vi "printTSR.vi"(0 "reference in":refnum<class "excelFile.lvclass">, 1 "TSR_details":T1={"Company/Institution:"="", "Address:"="", "Department:"="", "City:"="", "Post Code:"="", "Country:"="", "Contact:"="", "Ref:"="", "Issue description:"="", "Actions:"="", "TYPE:"="Repair", "Shipping:"=0, "Discount:"=0, "dataIN"=[], "Device type:"="microQuark", "Serial Number:"="", "PMC number:"="", "Labour Hours:"=0.0, "Service Location:"=FALSE, "start_hour"="", "end_hour"=""}, 3 "latest_TSR_path":string, 5 "error in (no error)":errorcluster) -> (14 "reference out":refnum<class "excelFile.lvclass">, 17 "PDF_file_path":string, 19 "error out":errorcluster)   [LabVIEW 2015, in "excelFile.lvclass"]
uses:
  excelFile.lvclass
  <vilib>/Utility/error.llb/DialogType.ctl
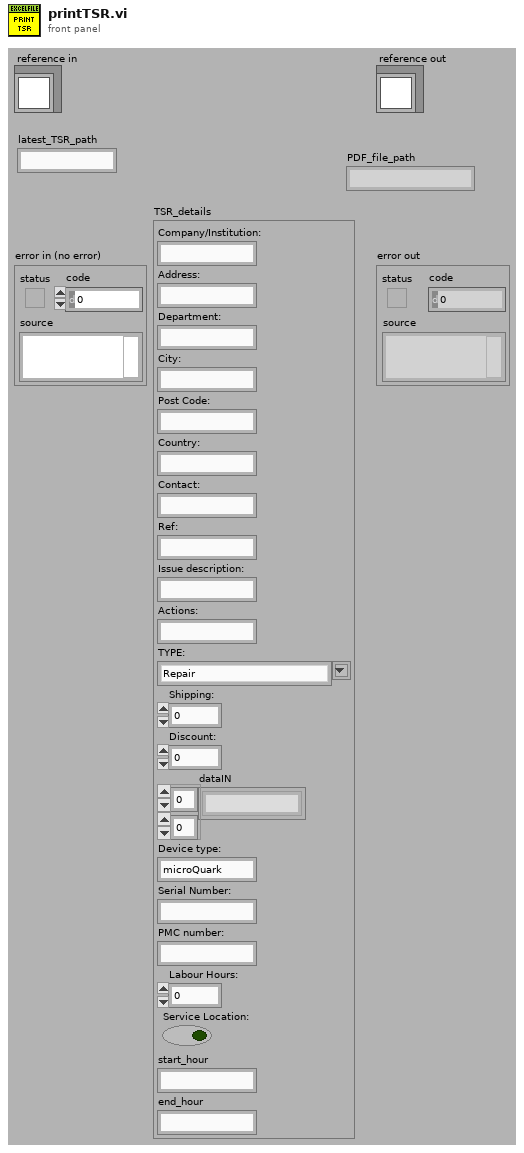
[diagram p1: front panel]
types:
  T1 = cluster{"Company/Institution:":string, "Address:":string, "Department:":string, "City:":string, "Post Code:":string, "Country:":string, "Contact:":string, "Ref:":string, "Issue description:":string, "Actions:":string, "TYPE:":string, "Shipping:":i32, "Discount:":i32, "dataIN":string[][], "Device type:":string, "Serial Number:":string, "PMC number:":string, "Labour Hours:":dbl, "Service Location:":bool, "start_hour":string, "end_hour":string}
  T2 = typedef "excelFile.lvclass/ObjectAttributesRef.ctl" = refnum<data-value>
  T3 = typedef "excelFile.lvclass/ObjectAttributes.ctl" = cluster{"MyAttribute":dbl, "path":string, "Refnum Excel":cluster{"Excel._Application":refnum<k7>, "Workbooks":refnum<k7>, "Open":refnum<k7>}, "data":string[][][], "save":bool, "fileType":T4, "rowsColor":u32[], "python_ref":refnum<class "python.lvclass">, "items_rows":i32[], "excel_range":i32[][], "TSR":cluster{"number":string, "TSR_path":path, "service_path":path, "email_to":string}, "excel_already_opened?":bool, "file_already_opened?":bool, "excel_protected_opened?":bool}
  T4 = typedef "excelFile.lvclass/fileType.ctl" = enum16{"devices", "items", "partsTracking", "TSR"}
  T5 = typedef "DialogType.ctl" = u16
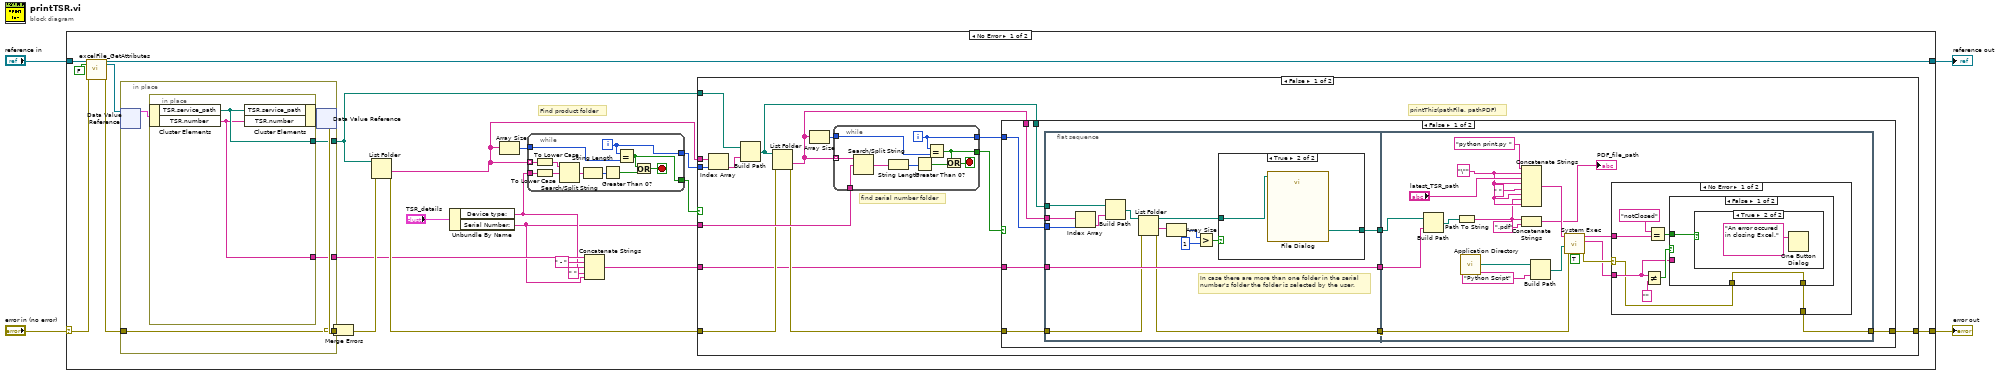
[diagram p0: block diagram]
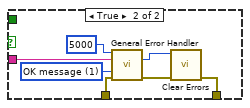
[diagram p4: hidden frame]
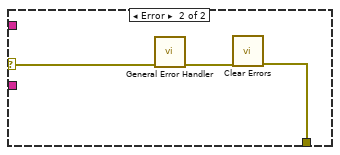
[diagram p5: hidden frame]
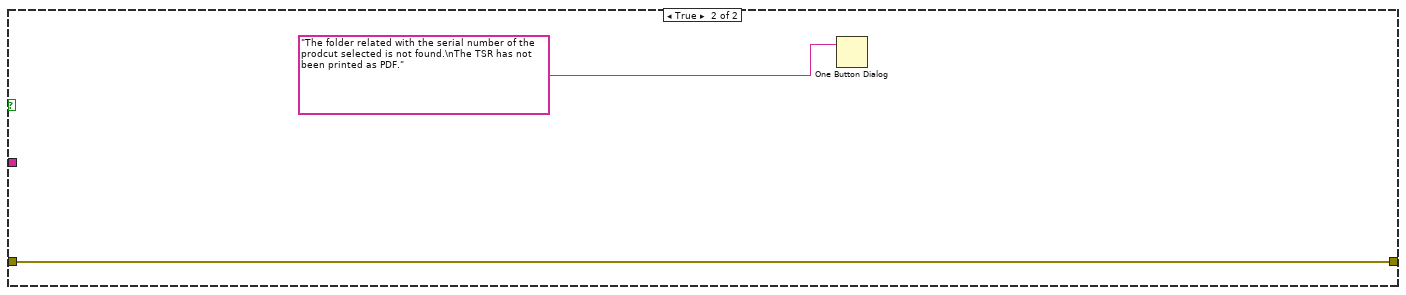
[diagram p6: hidden frame]
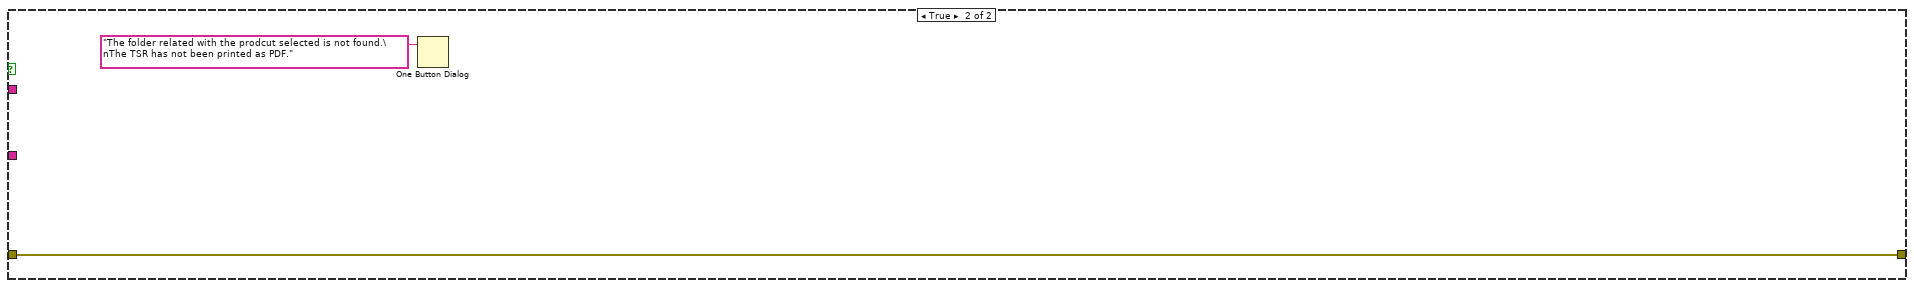
[diagram p7: hidden frame]
diagram:
  n1 = case shown="No Error" "error in (no error)" {
    selector: "error in (no error)" -> [w23 w141]
    tunnel: [w19 w141] -> w3
    tunnel: [w21 w140] -> w1
    tunnel: "reference in" -> [w25 w140]
    frame No Error {
      # "Find product folder"
      n2 = call "excelFile_GetAttributes.vi"("reference in"=w25, "return data? (T)"=FALSE, "error in (no error)"=w23) -> ("reference out"=w21:refnum<class "excelFile.lvclass">, "attributes ref"=w20:T2, "error out"=w22:errorcluster)  [unwired: 13 in, 1 out]
      n3 = in-place {
        in-place-border: w22 -> [w135]
        in-place-border: [w135] -> w26
        in-place-border: [w134] -> w18
        in-place-border: [w133] -> w11
        n4 = in-place-dvr #1(w20) -> (w136:T3)  [unwired: 1 out]
        n5 = in-place {
          in-place-border: [w139] -> w134
          in-place-border: [w138] -> w133
          n6 = in-place-cluster #2(w136) -> ("TSR.service_path"=w139:path, "TSR.number"=w138:string)
          n7 = in-place-cluster #2("TSR.service_path"=w139, "TSR.number"=w138) -> (w137:T3)
        }
        n8 = in-place-dvr #1(w137) -> (w27:errorcluster)  [unwired: 1 out]
      }
      n9 = Merge Errors(w26, w27) -> (w13:errorcluster)
      n10 = List Folder(path=w18, error in=w13) -> (folder names=w16:string[], error out=w14:errorcluster)  [unwired: 2 in, 2 out]
      n11 = Unbundle By Name("TSR_details") -> ("Device type:"=w9:string, "Serial Number:"=w6:string)
      n12 = Array Size(array=w16) -> (size(s)=w15:i32)
      n13 = while {
        tunnel: w16 -> [w130] mode=indexing
        tunnel: w9 -> [w128]
        tunnel: [w125] -> w17
        tunnel: w15 -> [w126]
        tunnel: [w122] -> w12
        i -> [w125]
        stop <- w123 stop-if-true
        n14 = To Lower Case(string=w130) -> (all lower case string=w129:string)
        n15 = To Lower Case(string=w128) -> (all lower case string=w127:string)
        n16 = Search/Split String(string=w129, search string/char (-)=w127) -> (match + rest of string=w132:string)  [unwired: 1 in, 2 out]
        n17 = String Length(string=w132) -> (length=w131:i32)
        n18 = Greater Than 0?(x=w131) -> (x > 0?=w124:bool)
        n19 = Equal?(x=w125, y=w126) -> (x = y?=w122:bool)
        n20 = Or(x=w122, y=w124) -> (x .or. y?=w123:bool)
      }
      n21 = Concatenate Strings(w11, " - " ("string"), w9, " " ("string"), w6) -> (w8:string)
      n22 = case shown="False" w12 {
        tunnel: [w41 w121] -> w19
        tunnel: w18 -> [w40 _]
        tunnel: w17 -> [w39 _]
        tunnel: w16 -> [w37 _]
        tunnel: w6 -> [w36 _]
        tunnel: w14 -> [w34 w121]
        tunnel: w8 -> [w32 _]
        frame False {
          # "find serial number folder"
          # "printThis(pathFile, pathPDF)"
          n23 = Index Array(array=w37, index=w39) -> (element=w38:string)
          n24 = Build Path(base path=w40, name or relative path=w38) -> (appended path=w30:path)
          n25 = List Folder(path=w30, error in=w34) -> (folder names=w29:string[], error out=w35:errorcluster)  [unwired: 2 in, 2 out]
          n26 = Array Size(array=w29) -> (size(s)=w28:i32)
          n27 = while {
            tunnel: [w115] -> w31
            tunnel: w29 -> [w117] mode=indexing
            tunnel: w36 -> [w116]
            tunnel: [w112] -> w33
            tunnel: w28 -> [w111]
            i -> [w115]
            stop <- w113 stop-if-true
            n28 = Search/Split String(string=w117, search string/char (-)=w116) -> (match + rest of string=w119:string)  [unwired: 1 in, 2 out]
            n29 = String Length(string=w119) -> (length=w118:i32)
            n30 = Greater Than 0?(x=w118) -> (x > 0?=w114:bool)
            n31 = Equal?(x=w115, y=w111) -> (x = y?=w112:bool)
            n32 = Or(x=w112, y=w114) -> (x .or. y?=w113:bool)
          }
          n33 = case shown="False" w33 {
            tunnel: [w46 w109] -> w41
            tunnel: w31 -> [w50 _]
            tunnel: w30 -> [w49 _]
            tunnel: w29 -> [w48 _]
            tunnel: w35 -> [w47 w109]
            tunnel: w32 -> [w45 _]
            frame False {
              n34 = flat-sequence {
                tunnel: w45 -> [w64]
                tunnel: w47 -> [w58]
                tunnel: w48 -> [w61]
                tunnel: w49 -> [w62]
                tunnel: w50 -> [w60]
                tunnel: [w57] -> w44
                tunnel: [w64] -> w43
                tunnel: [w53] -> w42
                tunnel: [w77] -> w46
                tunnel: w44 -> [w83]
                tunnel: w43 -> [w75]
                tunnel: w42 -> [w74]
                frame #0 {
                  # "In case there are more than one folder in the serial\nnumber's folder the folder is selected by the user."
                  n35 = Index Array(array=w61, index=w60) -> (element=w63:string)
                  n36 = Build Path(base path=w62, name or relative path=w63) -> (appended path=w59:path)
                  n37 = List Folder(path=w59, error in=w58) -> (path out=w54:path, folder names=w52:string[], error out=w57:errorcluster)  [unwired: 2 in, 1 out]
                  n38 = Array Size(array=w52) -> (size(s)=w51:i32)
                  n39 = Greater?(x=w51, y=1) -> (0:w55:bool)
                  n40 = case shown="True" w55 {
                    tunnel: w54 -> [w65 w67]
                    tunnel: [w65 w66] -> w53
                    frame False {
                    }
                    frame True {
                      n41 = call "File Dialog"("start path"=w67) -> ("selected path"=w66:path)  [unwired: 11 in, 3 out]
                    }
                  }
                }
                frame #1 {
                  w73 = "\"" ("string")
                  n42 = Build Path(base path=w74, name or relative path=w75) -> (appended path=w81:path)
                  n43 = Path To String(path=w81) -> (string=w72:string)
                  n44 = call <vilib>:"Application Directory.vi"() -> ("Application Directory"=w87:path)
                  n45 = Concatenate Strings("python print.py " ("command line"), w73, "latest_TSR_path", w73, " " ("string"), w73, w72, w73) -> (w79:string)
                  n46 = Concatenate Strings(w72, ".pdf" ("string")) -> (→"PDF_file_path":string)
                  n47 = Build Path(base path=w87, name or relative path="Python Script" ("string")) -> (appended path=w85:path)
                  n48 = call <vilib>:"System Exec.vi"("run minimized? (F)"=TRUE, "error in (no error)"=w83, "working directory"=w85, "command line"=w79) -> ("error out"=w78:errorcluster, "standard error"=w69:string, "standard output"=w68:string)  [unwired: 2 in, 3 out]
                  n49 = case shown="No Error" w78 {
                    selector: w78 -> [w92 w108]
                    tunnel: w69 -> [w93 _]
                    tunnel: [w91 w106] -> w77
                    tunnel: w68 -> [w90 _]
                    frame No Error {
                      n50 = Not Equal?(x=w93, y="") -> (x != y?=w94:bool)
                      n51 = Equal?(x="notClosed", y=w90) -> (x = y?=w88:bool)
                      n52 = case shown="False" w94 {
                        tunnel: w93 -> [_ w105]
                        tunnel: w92 -> [w97 w102]
                        tunnel: [w97 w100] -> w91
                        tunnel: w88 -> [w96 _]
                        frame False {
                          n53 = case shown="True" w96 {
                            frame False {
                            }
                            frame True {
                              n54 = One Button Dialog(message="An error occured in closing Excel.") -> ()  [unwired: 1 in, 1 out]
                            }
                          }
                        }
                        frame True {
                          w103 = T5 1 items=["no dialog", "OK message", "continue or stop message", "OK message + warnings", "continue/stop + warnings"] ("type of dialog (OK msg:1)")
                          n55 = call <vilib>:"General Error Handler.vi"("[error code] (0)"=5000, "[error source] (\" \")"=w105, "type of dialog (OK msg:1)"=w103, "error in (no error)"=w102) -> ("code out"=w99:i32, "error out"=w101:errorcluster)  [unwired: 7 in, 3 out]
                          n56 = call <vilib>:"Clear Errors.vi"("error in (no error)"=w101, "specific error code to clear (0: all)"=w99) -> ("error out"=w100:errorcluster)  [unwired: 4 in, 1 out]
                        }
                      }
                    }
                    frame Error {
                      n57 = call <vilib>:"General Error Handler.vi"("error in (no error)"=w108) -> ("error out"=w107:errorcluster)  [unwired: 10 in, 4 out]
                      n58 = call <vilib>:"Clear Errors.vi"("error in (no error)"=w107) -> ("error out"=w106:errorcluster)  [unwired: 5 in, 1 out]
                    }
                  }
                }
              }
            }
            frame True {
              n59 = One Button Dialog(message="The folder related with the serial number of the prodcut selected is not found.\nThe TSR has not been printed as PDF.") -> ()  [unwired: 1 in, 1 out]
            }
          }
        }
        frame True {
          n60 = One Button Dialog(message="The folder related with the prodcut selected is not found.\nThe TSR has not been printed as PDF.") -> ()  [unwired: 1 in, 1 out]
        }
      }
    }
    frame Error {
    }
  }
  "error out" <- w3
  "reference out" <- w1
